vi "CtrlTreeSaveState.vi"(8 "error in (no error)":errorcluster, 11 "TreeControl in":refnum<vi>) -> (0 "error out":errorcluster, 2 "State":T1, 3 "TreeControl out":refnum<vi>)   [LabVIEW 2021]
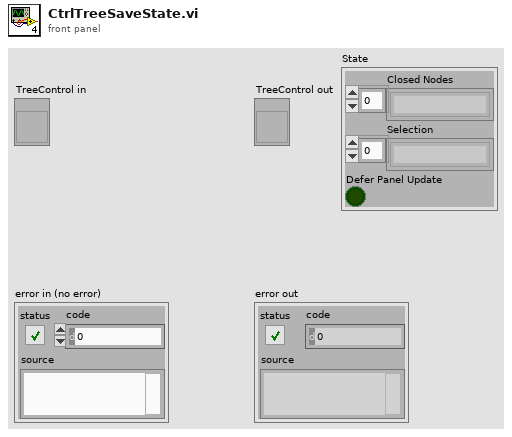
[diagram p1: front panel]
types:
  T1 = cluster{"Closed Nodes":string[], "Selection":string[], "Defer Panel Update":bool}
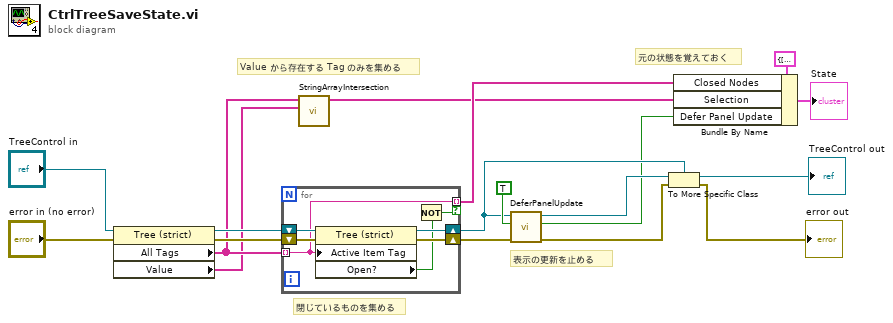
[diagram p0: block diagram]
diagram:
  # "元の状態を覚えておく"
  # "表示の更新を止める"
  # "Value から存在する Tag のみを集める"
  # "閉じているものを集める"
  n1 = property class="Tree (strict)"(reference="TreeControl in", error in="error in (no error)") -> (reference out=w17:refnum<vi>, error out=w18:errorcluster, "All Tags"=w5:string[], "Value"=w4:string[])
  n2 = for {
    tunnel: w5 -> [w21] mode=indexing
    shift-right: [w23] -> w10
    shift-left: w17 -> [w25]
    shift-right: [w22] -> w11
    shift-left: w18 -> [w24]
    tunnel: [w21] -> w6 mode=indexing if=w19
    n3 = property class="Tree (strict)"(reference=w25, error in=w24, "Active Item Tag"=w21) -> (reference out=w23:refnum<vi>, error out=w22:errorcluster, "Open?"=w20:bool)
    n4 = Not(x=w20) -> (.not. x?=w19:bool)
  }
  n5 = call "StringArrayIntersection.vi"("Fewer"=w4, "More"=w5) -> ("Intersection"=w3:string[])  [unwired: 9 in]
  n6 = call "DeferPanelUpdate.vi"("error in (no error)"=w11, "Defer Panel Updates (T)"=TRUE ("Defer Panel Updates"), "Control in"=w10) -> ("error out"=w2:errorcluster, "Defer Panel Updates Old"=w7:bool, "Control out"=w14:refnum<vi>)  [unwired: 6 in]
  n7 = To More Specific Class(target class=w10, reference=w14, error in=w2) -> (specific class reference=→"TreeControl out":refnum<vi>, error out=→"error out":errorcluster)
  n8 = Bundle By Name(cluster=T1 {"Closed Nodes"=[], "Selection"=[], "Defer Panel Update"=TRUE} ("Cluster"), "Closed Nodes"=w6, "Selection"=w3, "Defer Panel Update"=w7) -> (→"State":T1)
